vi "Post-Build Action.vi"(5 "Files Generated by Build":path[](array[path]), 6 "Top Level/Always Included VIs":path[](array[path]), 7 "Destination Path":path, 8 "error in (no error)":errorcluster, 9 "Target Name":string, 10 "Build Specification Name":string, 11 "Project Path":path) -> (0 "error out":errorcluster)   [LabVIEW 2017]
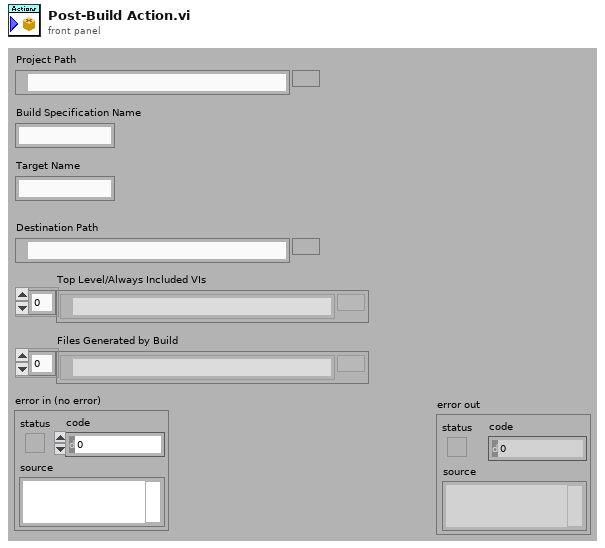
[diagram p1: front panel]
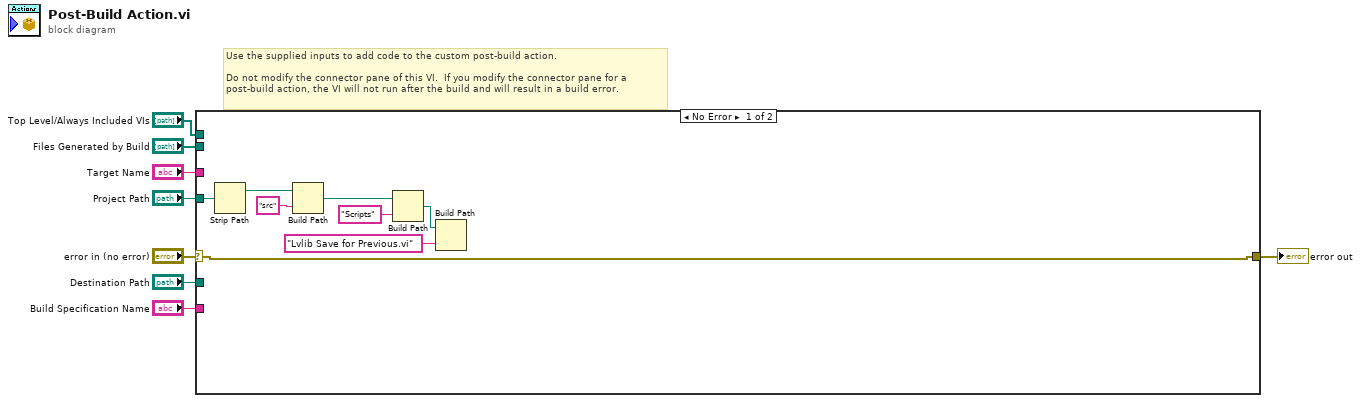
[diagram p0: block diagram]
diagram:
  # "Use the supplied inputs to add code to the custom post-build action.\n\nDo not modify the connector pane of this VI.  If you modify the connector pane for a post-build action, the VI will not run after the build and will result in a build error."
  n1 = case shown="No Error" "error in (no error)" {
    selector: "error in (no error)" -> [w9 w17]
    tunnel: [w9 w17] -> w8
    tunnel: "Destination Path" -> [_ _]
    tunnel: "Build Specification Name" -> [_ _]
    tunnel: "Project Path" -> [w11 _]
    tunnel: "Target Name" -> [_ _]
    tunnel: "Top Level/Always Included VIs" -> [_ _]
    tunnel: "Files Generated by Build" -> [_ _]
    frame No Error {
      n2 = Strip Path(path=w11) -> (stripped path=w10:path)  [unwired: 1 out]
      n3 = Build Path(base path=w10, name or relative path="src") -> (appended path=w15:path)
      n4 = Build Path(base path=w15, name or relative path="Scripts") -> (appended path=w13:path)
      n5 = Build Path(base path=w13, name or relative path="Lvlib Save for Previous.vi") -> ()  [unwired: 1 out]
    }
    frame Error {
    }
  }
  "error out" <- w8
